vi "sensor count.vi"(0 "sensor thr array":dbl[](array[numeric]), 1 "pallet speed":dbl=0.25 format="%#_13g", 2 "speed array in":dbl[](array[numeric]), 5 "capture y or no ?":bool, 7 "sensor data":dbl[](array[numeric]), 9 "counter input":i8, 11 "counting role":T1(ring), 12 "error in":errorcluster, 13 "falling level thr":dbl=59000.0 format="%#_13g") -> (3 "column count":bool, 4 "speed array out":dbl[](array[numeric]), 6 "sensor counter":bool, 8 "Elapsed Time (s)":dbl, 10 "counter out":i8, 14 "pallet detect":bool, 15 "error out":errorcluster)   [LabVIEW 2019]
uses:
  <vilib>/measure/mamon.llb/Trigger Detection for 1 Channel.vi
  <vilib>/measure/NI_MAPro.lvlib
panel:
  out "Numeric 3":i32=1
  out "Numeric 2":i32=1
  out "Numeric":i32=1
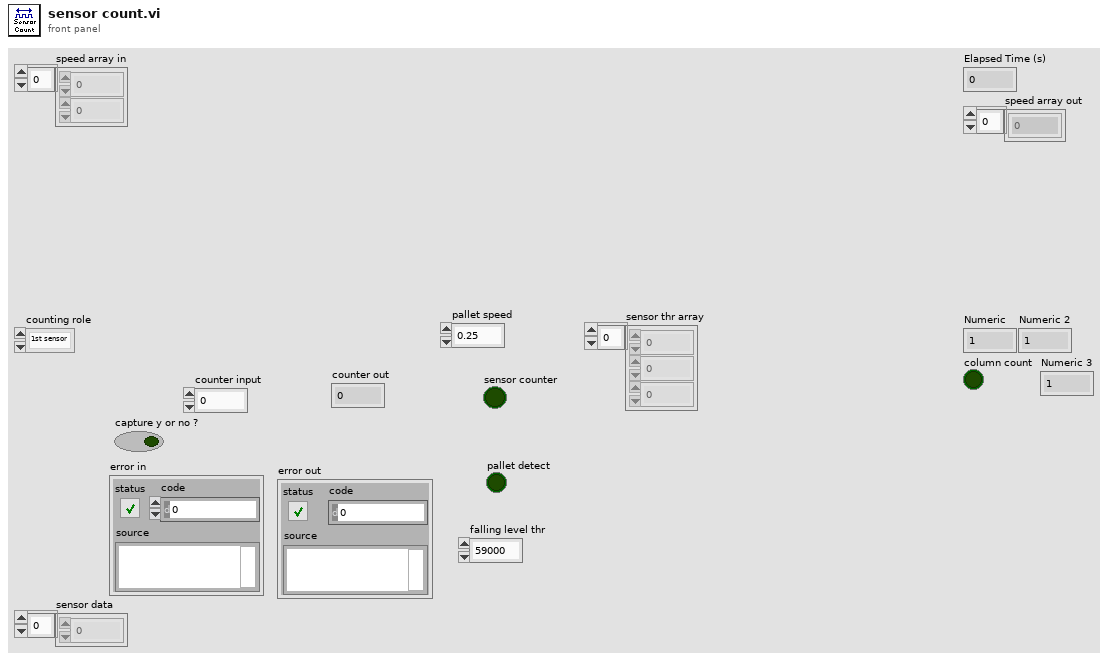
[diagram p1: front panel]
types:
  T1 = enum16{"1st sensor", "2nd sensor", "3rd sensor", "1st+2nd", "1st+3rd", "2nd+3rd", "1st+2nd+3rd"}
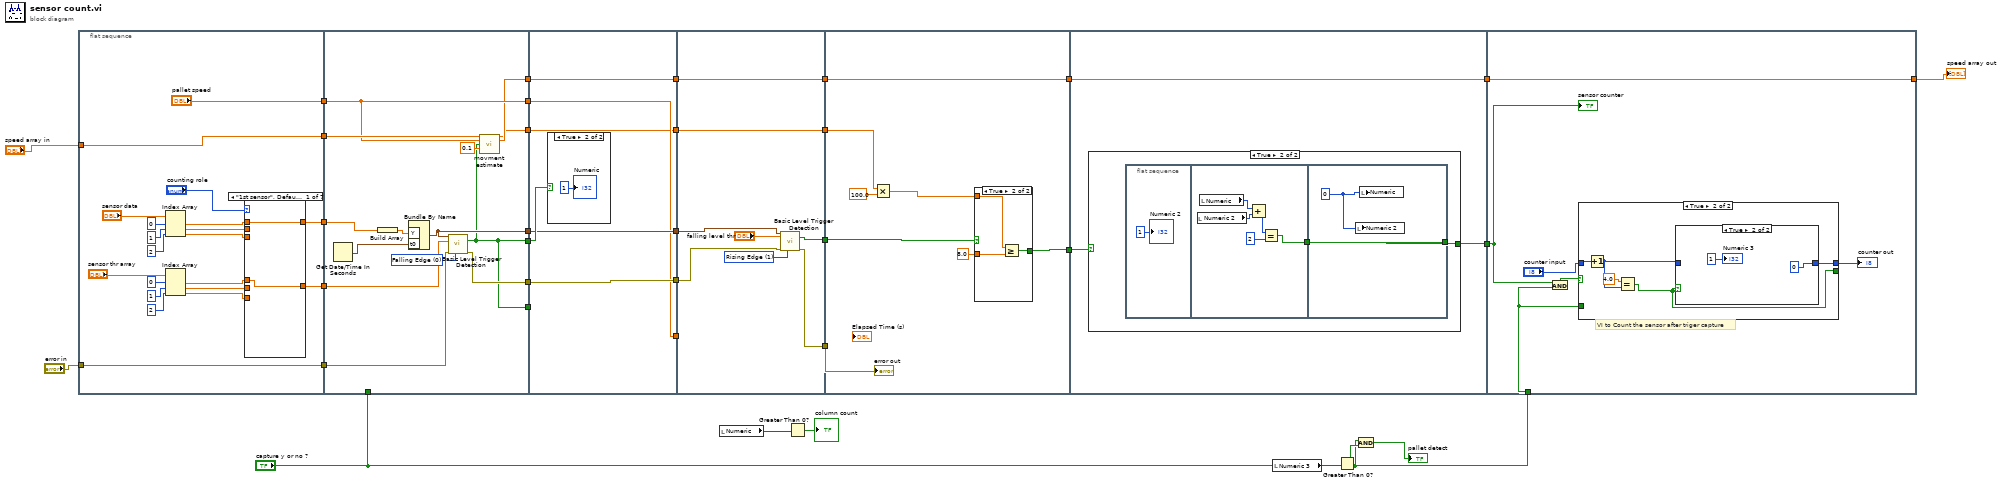
[diagram p0: block diagram]
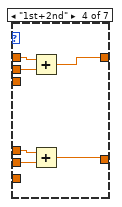
[diagram p4: hidden frame]
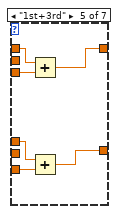
[diagram p5: hidden frame]
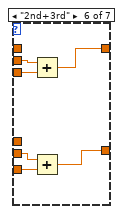
[diagram p6: hidden frame]
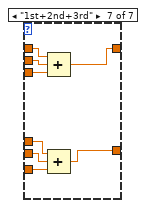
[diagram p7: hidden frame]
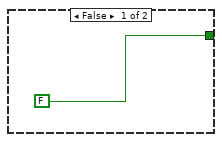
[diagram p10: hidden frame]
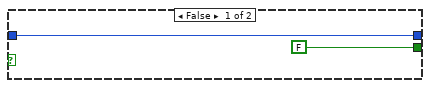
[diagram p11: hidden frame]
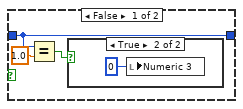
[diagram p12: hidden frame]
diagram:
  n1 = flat-sequence {
    tunnel: "error in" -> [w39]
    tunnel: [w39] -> w30
    tunnel: [w38] -> w29
    tunnel: [w37] -> w28
    tunnel: [w36] -> w16
    tunnel: "speed array in" -> [w36]
    tunnel: ["pallet speed"] -> w11
    tunnel: w30 -> [w100]
    tunnel: w29 -> [w94]
    tunnel: w28 -> [w93]
    tunnel: [w87] -> w27
    tunnel: [w99] -> w26
    tunnel: [w97] -> w24
    tunnel: w16 -> [w92]
    tunnel: [w87] -> w14
    tunnel: [w91] -> w12
    tunnel: w11 -> [w91]
    tunnel: "capture y or no ?" -> [_]
    tunnel: [w89] -> w4
    tunnel: [w88] -> w1
    tunnel: w27 -> [w106]
    tunnel: w26 -> [w104]
    tunnel: [w105] -> w25
    tunnel: w24 -> [w105]
    tunnel: [w104] -> w23
    tunnel: w14 -> [_]
    tunnel: [w103] -> w13
    tunnel: w12 -> [w103]
    tunnel: [w102] -> w5
    tunnel: w4 -> [w102]
    tunnel: [w101] -> w2
    tunnel: w1 -> [w101]
    tunnel: w25 -> [w113]
    tunnel: w23 -> [w112]
    tunnel: [w111] -> w22
    tunnel: [w110] -> w19
    tunnel: w13 -> [_]
    tunnel: [w109] -> w6
    tunnel: w5 -> [w109]
    tunnel: [w108] -> w3
    tunnel: w2 -> [w108]
    tunnel: w22 -> [w123]
    tunnel: [w122] -> w21
    tunnel: w19 -> [w121]
    tunnel: [w119] -> w7
    tunnel: w6 -> [w119]
    tunnel: w3 -> [w118]
    tunnel: w21 -> [w130]
    tunnel: [w129] -> w20
    tunnel: [w128] -> w8
    tunnel: w7 -> [w128]
    tunnel: "capture y or no ?" -> [w143]
    tunnel: w20 -> [w144]
    tunnel: [w142] -> w9
    tunnel: w8 -> [w142]
    frame #0 {
      n2 = Index Array(array="sensor data", index #1=0 ("index"), index #2=1 ("index"), index #3=2 ("index")) -> (element #1=w52:dbl, element #2=w53:dbl, element #3=w54:dbl)
      n3 = Index Array(array="sensor thr array", index #1=0 ("index"), index #2=1 ("index"), index #3=2 ("index")) -> (element #1=w48:dbl, element #2=w49:dbl, element #3=w50:dbl)
      n4 = case shown="\"1st sensor\", Default" "counting role" {
        tunnel: w52 -> [w56 _ _ w64 w72 _ w86]
        tunnel: w48 -> [w55 _ _ w65 w70 _ w83]
        tunnel: w53 -> [_ w58 _ w66 _ w78 w85]
        tunnel: w54 -> [_ _ w60 _ w71 w77 w84]
        tunnel: w49 -> [_ w57 _ w63 _ w76 w82]
        tunnel: w50 -> [_ _ w59 _ w69 w75 w81]
        tunnel: [w56 w58 w60 w62 w68 w74 w80] -> w38
        tunnel: [w55 w57 w59 w61 w67 w73 w79] -> w37
        frame "1st sensor", Default {
        }
        frame "2nd sensor" {
        }
        frame "3rd sensor" {
        }
        frame "1st+2nd" {
          n5 = Add(x=w64, y=w66) -> (x+y=w62:dbl)
          n6 = Add(x=w65, y=w63) -> (x+y=w61:dbl)
        }
        frame "1st+3rd" {
          n7 = Add(x=w72, y=w71) -> (x+y=w68:dbl)
          n8 = Add(x=w70, y=w69) -> (x+y=w67:dbl)
        }
        frame "2nd+3rd" {
          n9 = Add(x=w78, y=w77) -> (x+y=w74:dbl)
          n10 = Add(x=w76, y=w75) -> (x+y=w73:dbl)
        }
        frame "1st+2nd+3rd" {
          n11 = Compound Arithmetic op=ADD(w86, w85, w84) -> (w80:dbl)
          n12 = Compound Arithmetic op=ADD(w83, w82, w81) -> (w79:dbl)
        }
      }
    }
    frame #1 {
      w95 = u16 0 items=["Falling Edge", "Rising Edge"] ("trigger slope")
      n13 = Get Date/Time In Seconds() -> (seconds since 1Jan1904=w96:timestamp)
      n14 = Build Array(w94) -> (w98:dbl[])
      n15 = Bundle By Name("Y"=w98, "t0"=w96) -> (w97:waveform(dbl))  [unwired: 1 in]
      n16 = call-poly <vilib>:"Basic Level Trigger Detection.vi"("signal in"=w97, "level"=w93, "error in (no error)"=w100, "trigger slope"=w95) -> ("trigger detected?"=w87:bool, "error out"=w99:errorcluster)  [unwired: 9 in, 1 out]
      n17 = call "movment estimate.vi"("speed array in"=w92, "speed"=w91, "start"=w87, "speed limit change"=0.1) -> ("total movement"=w88:dbl, "speed array out"=w89:dbl[])  [unwired: 10 in]
    }
    frame #2 {
      n18 = case shown="True" w106 {
        frame False {
        }
        frame True {
          "Numeric" <- 1
        }
      }
    }
    frame #3 {
      w114 = u16 1 items=["Falling Edge", "Rising Edge"] ("trigger slope")
      n19 = call-poly <vilib>:"Basic Level Trigger Detection.vi"("signal in"=w113, "level"="falling level thr", "error in (no error)"=w112, "trigger slope"=w114) -> ("trigger detected?"=w111:bool, "error out"=w110:errorcluster)  [unwired: 9 in, 1 out]
    }
    frame #4 {
      n20 = Multiply(x=w118, y=100.0) -> (x*y=w116:dbl)
      n21 = case shown="True" w123 {
        selector: w123 -> [w124 _]
        tunnel: [w124 w127] -> w122
        tunnel: 8.0 -> [_ w126]
        tunnel: w116 -> [_ w125]
        frame False {
        }
        frame True {
          n22 = Greater Or Equal?(x=w125, y=w126) -> (x >= y?=w127:bool)
        }
      }
      "error out" <- w121
    }
    frame #5 {
      n23 = case shown="True" w130 {
        tunnel: [FALSE w133] -> w129
        frame False {
        }
        frame True {
          n24 = flat-sequence {
            tunnel: [w135] -> w132
            tunnel: [w141] -> w133
            tunnel: w132 -> [w141]
            frame #0 {
              "Numeric 2" <- 1
            }
            frame #1 {
              n25 = local read "Numeric 2"() -> (w138:i32)
              n26 = local read "Numeric"() -> (w139:i32)
              n27 = Add(x=w139, y=w138) -> (x+y=w137:i32)
              n28 = Equal?(x=w137, y=2) -> (x = y?=w135:bool)
            }
            frame #2 {
              w140 = 0 ("Numeric")
              n29 = local write "Numeric 2"(w140) -> ()
              n30 = local write "Numeric"(w140) -> ()
            }
          }
        }
      }
    }
    frame #6 {
      # "VI to Count the sensor after triger capture"
      n31 = And(x=w144, y=w143) -> (x .and. y?=w147:bool)
      n32 = case shown="True" w147 {
        tunnel: "counter input" -> [w149 w153]
        tunnel: [w149 w151] -> w145
        tunnel: [FALSE w150] -> _
        tunnel: w143 -> [_ _]
        frame False {
        }
        frame True {
          n33 = Increment(x=w153) -> (x+1=w152:i8)
          n34 = Equal?(x=4.0, y=w152) -> (x = y?=w150:bool)
          n35 = case shown="True" w150 {
            tunnel: w152 -> [w157 _]
            tunnel: [w157 i8 0 ("counter out")] -> w151
            frame False {
              n36 = Equal?(x=w157, y=1.0) -> (x = y?=w155:bool)
              n37 = case shown="True" w155 {
                frame False {
                }
                frame True {
                  n38 = local write "Numeric 3"(0 ("Numeric 3")) -> ()
                }
              }
            }
            frame True {
              "Numeric 3" <- 1
            }
          }
        }
      }
      "counter out" <- w145
      "sensor counter" <- w144
    }
  }
  n39 = local read "Numeric"() -> (w34:i32)
  n40 = Greater Than 0?(x=w34) -> (x > 0?=→"column count":bool)
  n41 = local read "Numeric 3"() -> (w32:i32)
  n42 = Greater Than 0?(x=w32) -> (x > 0?=w18:bool)
  n43 = And(x="capture y or no ?", y=w18) -> (x .and. y?=→"pallet detect":bool)
  "speed array out" <- w9
